vi "Write Drive Sensors.vi"(8 "error in (no error)":errorcluster, 10 "Drive Sensors":T1, 11 "Drive in":refnum<class "Drive.lvclass">) -> (0 "error out":errorcluster, 3 "Drive out":refnum<class "Drive.lvclass">)   [LabVIEW 2018, in "Drive.lvlib" / "Drive.lvclass"]
uses:
  Drive.lvclass
  Controls/Drive Sensor Data.ctl
  Drive.lvclass/Drive.ctl
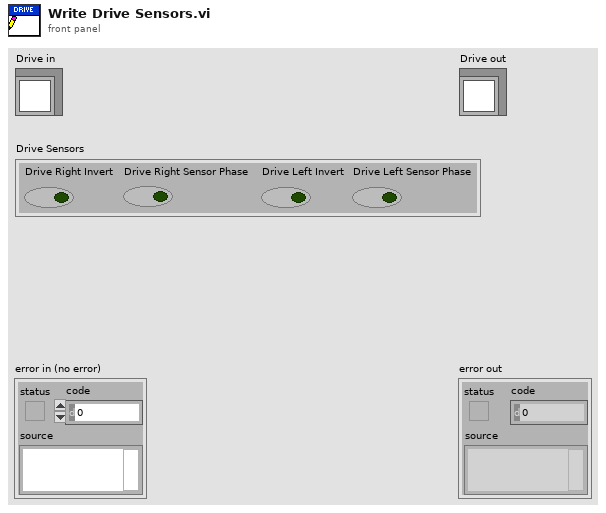
[diagram p1: front panel]
types:
  T1 = typedef "Drive.lvlib/Drive.lvclass/Drive Sensor Data.ctl" = cluster{"Drive Right Invert":bool, "Drive Right Sensor Phase":bool, "Drive Left Invert":bool, "Drive Left Sensor Phase":bool}
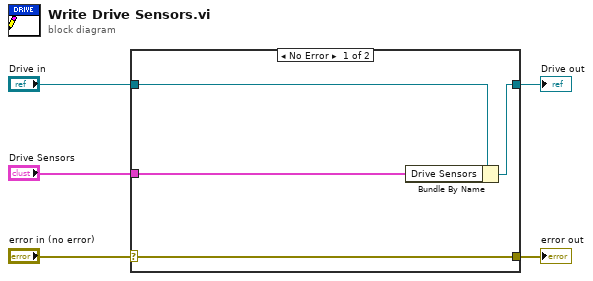
[diagram p0: block diagram]
diagram:
  n1 = case shown="No Error" "error in (no error)" {
    selector: "error in (no error)" -> [w9 w10]
    tunnel: [w9 w10] -> w4
    tunnel: [w7 w11] -> w2
    tunnel: "Drive in" -> [w8 w11]
    tunnel: "Drive Sensors" -> [w6 _]
    frame No Error {
      n2 = Bundle By Name(cluster=w8, "Drive Sensors"=w6) -> (w7:refnum<class "Drive.lvclass">)
    }
    frame Error {
    }
  }
  "error out" <- w4
  "Drive out" <- w2
